vi "MakeButtonsAndLinks.vi"(9 "Simplified":bool, 11 "Nagivations":T1[](array[typedef])) -> (2 "Links":string, 3 "Buttons":string)   [LabVIEW 2021, in "ButtonBarFlow.lvlib"]
uses:
  ButtonBarFlow.lvlib
  ActiveObjects/VerticalButtonBar/ButtonCollection/ButtonDefinition.ctl
  ActiveObjects/VerticalButtonBar/ButtonCollection/ButtonCollection.lvclass
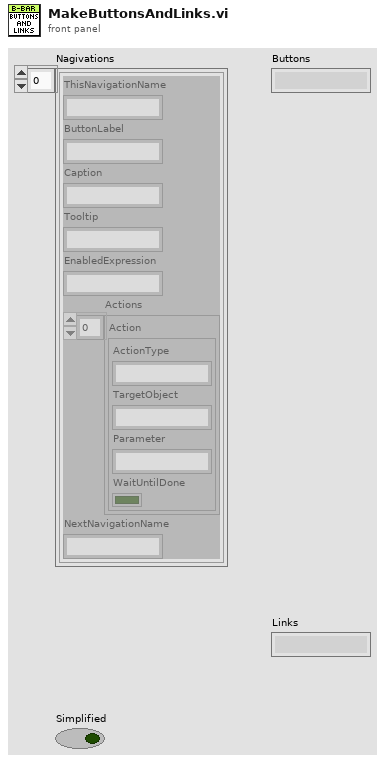
[diagram p1: front panel]
types:
  T1 = typedef "ButtonCollection.lvclass/ButtonDefinition.ctl" = cluster{"ThisNavigationName":string, "ButtonLabel":string, "Caption":string, "Tooltip":string, "EnabledExpression":string, "Actions":cluster{"ActionType":string, "TargetObject":string, "Parameter":string, "WaitUntilDone":bool}[], "NextNavigationName":string}
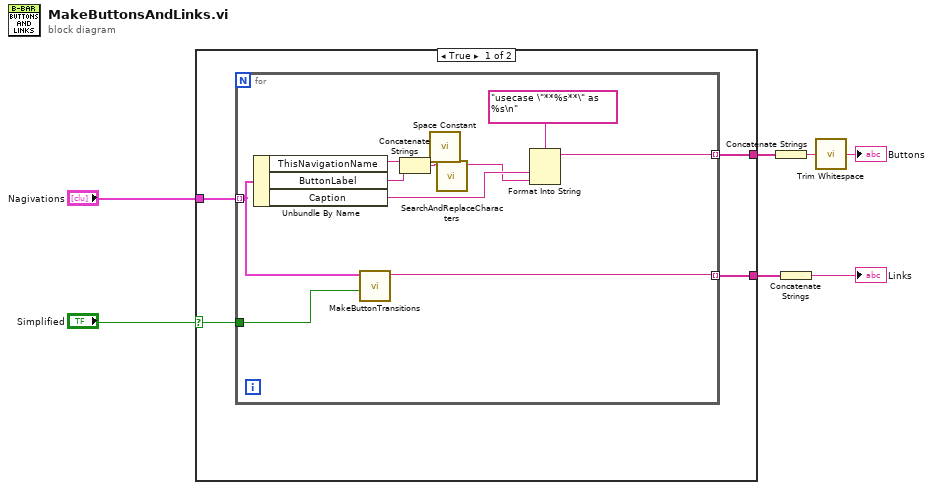
[diagram p0: block diagram]
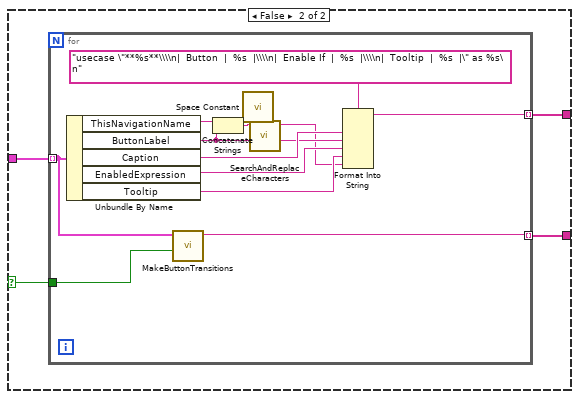
[diagram p2: hidden frame]
diagram:
  n1 = case shown="True" "Simplified" {
    selector: "Simplified" -> [w8 w23]
    tunnel: "Nagivations" -> [w11 w26]
    tunnel: [w10 w25] -> w6
    tunnel: [w9 w24] -> w4
    frame True {
      n2 = for {
        tunnel: w11 -> [w14] mode=indexing
        tunnel: [w13] -> w9 mode=indexing
        tunnel: [w20] -> w10 mode=indexing
        tunnel: w8 -> [w12]
        n3 = Unbundle By Name(w14) -> ("ThisNavigationName"=w21:string, "ButtonLabel"=w18:string, "Caption"=w19:string)
        n4 = call "MakeButtonTransitions.vi"("Simplified"=w12, "NavigationItem"=w14) -> ("PlantUML"=w13:string)  [unwired: 9 in]
        n5 = Concatenate Strings(w21, w18) -> (w16:string)
        n6 = call <vilib>:"Space Constant.vi"() -> ("String"=w17:string)
        n7 = call "SearchAndReplaceCharacters.vi"("CharactersToSearch"=w17, "StringIn"=w16) -> ("ResultString"=w15:string)  [unwired: 9 in]
        n8 = Format Into String(format string="usecase \"**%s**\" as %s\n", w19, w15) -> (resulting string=w20:string)  [unwired: 2 in, 1 out]
      }
    }
    frame False {
      n9 = for {
        tunnel: w26 -> [w29] mode=indexing
        tunnel: [w28] -> w24 mode=indexing
        tunnel: [w37] -> w25 mode=indexing
        tunnel: w23 -> [w27]
        n10 = Unbundle By Name(w29) -> ("ThisNavigationName"=w38:string, "ButtonLabel"=w33:string, "Caption"=w34:string, "EnabledExpression"=w36:string, "Tooltip"=w35:string)
        n11 = call "MakeButtonTransitions.vi"("Simplified"=w27, "NavigationItem"=w29) -> ("PlantUML"=w28:string)  [unwired: 9 in]
        n12 = Concatenate Strings(w38, w33) -> (w31:string)
        n13 = call <vilib>:"Space Constant.vi"() -> ("String"=w32:string)
        n14 = call "SearchAndReplaceCharacters.vi"("CharactersToSearch"=w32, "StringIn"=w31) -> ("ResultString"=w30:string)  [unwired: 9 in]
        n15 = Format Into String(format string="usecase \"**%s**\\\\n|  Button  |  %s  |\\\\n|  Enable If  |  %s  |\\\\n|  Tooltip  |  %s  |\" as %s\n", w34, w33, w36, w35, w30) -> (resulting string=w37:string)  [unwired: 2 in, 1 out]
      }
    }
  }
  n16 = Concatenate Strings(w6) -> (w5:string)
  n17 = Concatenate Strings(w4) -> (→"Links":string)
  n18 = call <vilib>:"Trim Whitespace.vi"("string"=w5) -> ("trimmed string"=→"Buttons":string)  [unwired: 1 in]
